vi "USER_EDITOR_scan_barcode.vi"(8 "error_in":errorcluster, 11 "all_config_info":T1={"main_ini_file"={"SQL Driver"="", "SQL Server"="", "SQL Database"="", "SQL UID"="", "Reference table"="", "Reference history"="", "Archivisation CFG table"="", "Archivisation CFG history"="", "User table"="", "User history"="", "logout timeout [ms]"=0, "records per page"=0, "default language"="", "REF CHG connection IP"="", "REF CHG remote port"=0, "REF CHG local port"=0, "SCANNER COM port"=0, "SCANNER Baud rate"=0, "SCANNER Data bits"=0, "SCANNER Pairity"=enum."None", "SCANNER Stop bits"=10, "SCANNER Flow control"=0, "SCANNER Termination char"=0}, "SQL Password"="", "queue_refnums"={"SQL_EDITOR_queue"=refnum, "SCANNER_queue"=refnum, "SCANNER_data"=refnum, "CLIENT_REF_CHG_queue"=refnum}} {"main_ini_file"."SCANNER Flow control" items=["None"=0, "XON/XOFF"=1, "RTS/CTS"=2, "DTR/DSR"=4]; "main_ini_file"."SCANNER Stop bits" items=["1.0"=10, "1.5"=15, "2.0"=20]}) -> (0 "error_out":errorcluster, 2 "Canceled?":bool, 3 "barcode":string)   [LabVIEW 2019]
uses:
  ini/typedef/CLIENT_all_config_info.ctl
  ini/typedef/CLIENT_main_ini_file.ctl
  queues/typedef/CLIENT_queue_refnums.ctl
  queues/typedef/SQL_EDITOR_queue_element.ctl
  SQL_EDITOR/SQL_EDITOR_sequence_state.ctl
  queues/typedef/CLIENT_SCANNER_queue_element.ctl
  SCANNER/SCANNER_sequence_state.ctl
  queues/typedef/CLIENT_REF_CHG_queue_element.ctl
  reference_changed_connection/CLIENT_REF_CHG_sequence_state.ctl
panel:
  in  "cancel_barcode_scan":bool
  # "Waiting for barcode scan..."
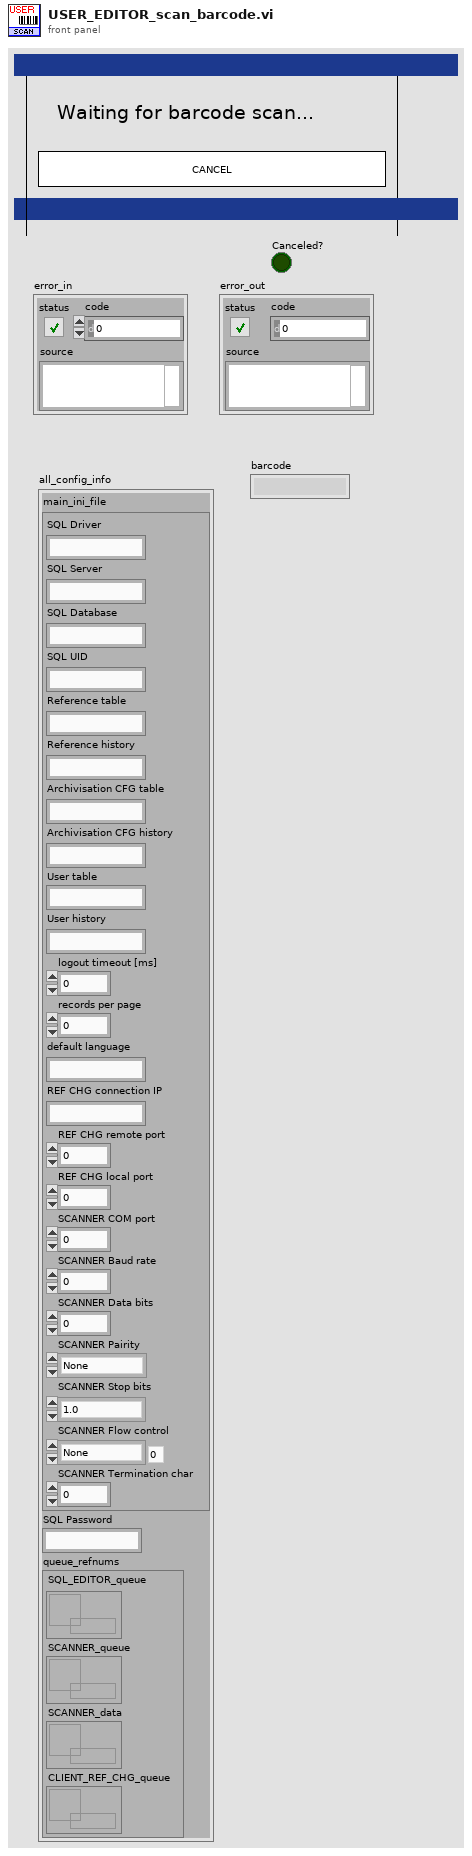
[diagram p1: front panel]
types:
  T1 = typedef "CLIENT_all_config_info.ctl" = cluster{"main_ini_file":T2, "SQL Password":string, "queue_refnums":T3}
  T2 = typedef "CLIENT_main_ini_file.ctl" = cluster{"SQL Driver":string, "SQL Server":string, "SQL Database":string, "SQL UID":string, "Reference table":string, "Reference history":string, "Archivisation CFG table":string, "Archivisation CFG history":string, "User table":string, "User history":string, "logout timeout [ms]":i32, "records per page":i32, "default language":string, "REF CHG connection IP":string, "REF CHG remote port":i32, "REF CHG local port":i32, "SCANNER COM port":u16, "SCANNER Baud rate":u32, "SCANNER Data bits":u16, "SCANNER Pairity":enum16{"None", "Odd", "Even", "Mark", "Space"}, "SCANNER Stop bits":u16, "SCANNER Flow control":u16, "SCANNER Termination char":u8}
  T3 = typedef "CLIENT_queue_refnums.ctl" = cluster{"SQL_EDITOR_queue":refnum<queue>, "SCANNER_queue":refnum<queue>, "SCANNER_data":refnum<queue>, "CLIENT_REF_CHG_queue":refnum<queue>}
  T4 = typedef "CLIENT_SCANNER_queue_element.ctl" = cluster{"state":T5, "variable":variant}
  T5 = typedef "SCANNER_sequence_state.ctl" = enum16{"initialize", "get_next_state", "read", "cancel_read", "error", "stop"}
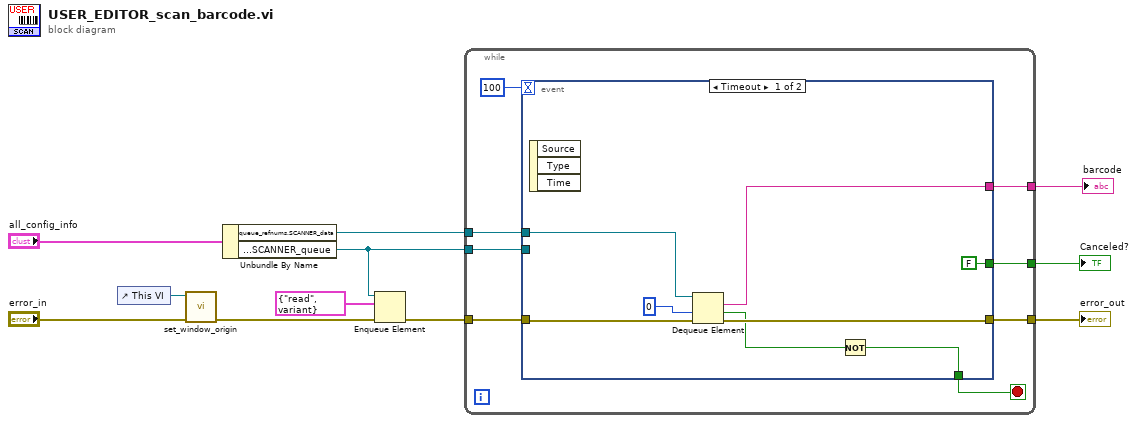
[diagram p0: block diagram]
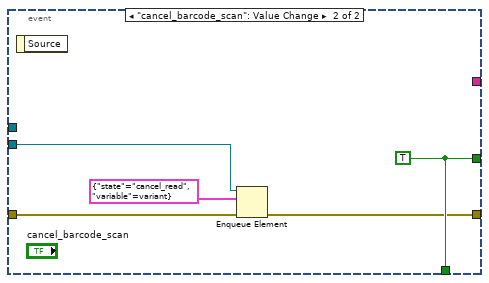
[diagram p2: hidden frame]
diagram:
  n1 = control-ref of="This VI"() -> (w10:refnum<vi>)
  n2 = call "set_window_origin.vi"("error_in"="error_in", "this_vi_reference"=w10) -> ("error_out"=w5:errorcluster)  [unwired: 9 in]
  n3 = Unbundle By Name("all_config_info") -> ("queue_refnums.SCANNER_data"=w7:refnum<queue>, "queue_refnums.SCANNER_queue"=w1:refnum<queue>)
  n4 = Enqueue Element(queue=w1, element=T4 {"state"=enum."read", "variable"=variant}, error in (no error)=w5) -> (error out=w4:errorcluster)  [unwired: 1 in, 2 out]
  n5 = while {
    tunnel: w4 -> [w19]
    tunnel: [w18] -> w11
    tunnel: w7 -> [w16]
    tunnel: [w15] -> w6
    tunnel: [w13] -> w2
    tunnel: w1 -> [w12]
    stop <- w14 stop-if-true
    n6 = event shown="[0] Timeout" {
      selector: _ -> [_ _]
      dyn-events: _ -> [_ _]
      timeout: 100 -> [_ _]
      tunnel: w19 -> [w26 w31]
      tunnel: [w25 w28] -> w18
      tunnel: [w21 w32] -> w14
      tunnel: w16 -> [w27 _]
      tunnel: [w22 _] -> w15
      tunnel: [FALSE w32] -> w13
      tunnel: w12 -> [_ w30]
      event Timeout {
        n7 = event-data() -> ()  [unwired: 1 in, 3 out]
        n8 = Dequeue Element(queue=w27, timeout in ms (-1)=0, error in (no error)=w26) -> (element=w22:string, timed out?=w23:bool, error out=w25:errorcluster)  [unwired: 1 out]
        n9 = Not(x=w23) -> (.not. x?=w21:bool)
      }
      event "cancel_barcode_scan": Value Change {
        w32 = TRUE
        n10 = event-data() -> ()  [unwired: 1 in, 1 out]
        n11 = Enqueue Element(queue=w30, element=T4 {"state"=enum."cancel_read", "variable"=variant}, error in (no error)=w31) -> (error out=w28:errorcluster)  [unwired: 1 in, 2 out]
      }
    }
  }
  "error_out" <- w11
  "barcode" <- w6
  "Canceled?" <- w2
